vi "get execution system.vi"(11 "task in":refnum<class "task.lvclass">) -> (2 "execution system":T1, 3 "task out":refnum<class "task.lvclass">)   [LabVIEW 2013, in "task.lvclass"]
uses:
  task.lvclass
  dispatcher/execution system.ctl
  task.lvclass/task.ctl
  dispatcher/thread pool.lvclass
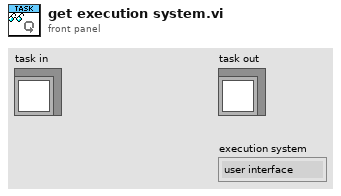
[diagram p1: front panel]
types:
  T1 = typedef "thread pool.lvclass/execution system.ctl" = enum32{"user interface", "standard", "instrument i/o", "data acquisition", "other 1", "other 2"}
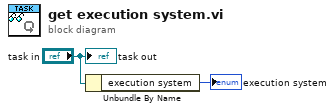
[diagram p0: block diagram]
diagram:
  n1 = Unbundle By Name("task in") -> ("execution system"=→"execution system":T1)
  "task out" <- "task in"
